vi "Generate Differential Drive Trajectory.vi"(8 "error in (no error)":errorcluster, 9 "Constraints":T1={"maxVoltage"=10.0, "maxVelocity"=5.0, "maxAccel"=10.0}, 10 "Constants":T2={"ks"=0.2, "kv"=0.18, "ka"=0.1, "trackwidth"=1.0}, 11 "Waypoints":T3[](array[typedef])=[{"Translation2d"={"x"=0.0, "y"=0.0}, "Rotation2d"={"Theta"=0.0}}, {"Translation2d"={"x"=1.0, "y"=1.0}, "Rotation2d"={"Theta"=1.0}}, {"Translation2d"={"x"=3.0, "y"=4.0}, "Rotation2d"={"Theta"=2.0}}]) -> (0 "error out":errorcluster, 2 "Total Time Seconds":dbl, 3 "states":T6[](array[typedef]))   [LabVIEW 2019]
uses:
  Typedef/Trajectory State.ctl
  Geometry/Typedef/Pose2d.ctl
  Geometry/Typedef/Translation2d.ctl
  Geometry/Typedef/Rotation2d.ctl
  Typedef/Differential Drive Constants.ctl
  Typedef/Differential Drive Constraints.ctl
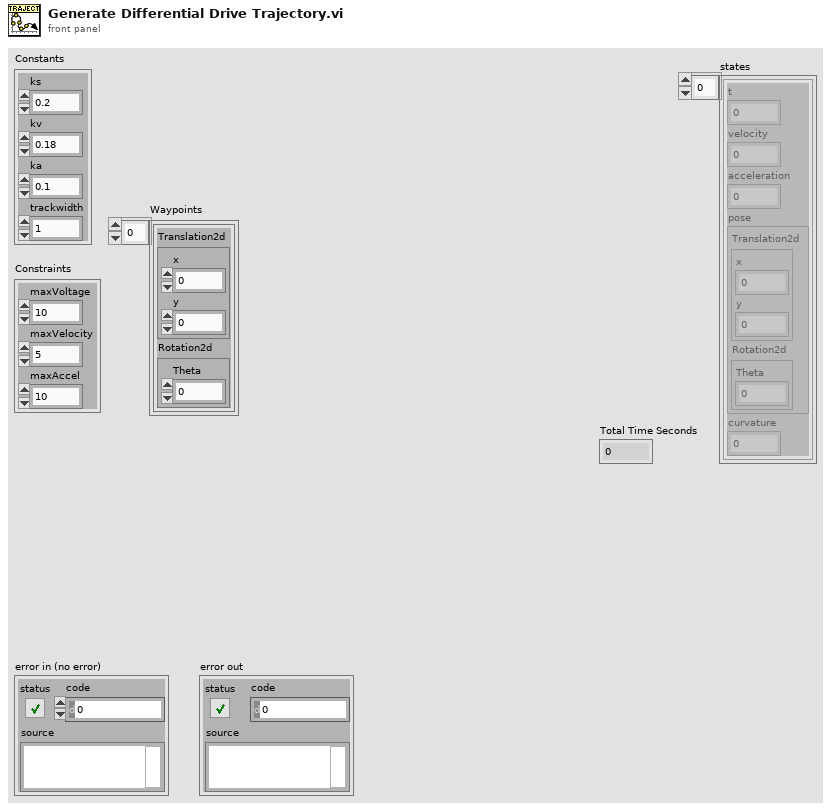
[diagram p1: front panel]
types:
  T1 = typedef "Differential Drive Constraints.ctl" = cluster{"maxVoltage":dbl, "maxVelocity":dbl, "maxAccel":dbl}
  T2 = typedef "Differential Drive Constants.ctl" = cluster{"ks":dbl, "kv":dbl, "ka":dbl, "trackwidth":dbl}
  T3 = typedef "Pose2d.ctl" = cluster{"Translation2d":T4, "Rotation2d":T5}
  T4 = typedef "Translation2d.ctl" = cluster{"x":dbl, "y":dbl}
  T5 = typedef "Rotation2d.ctl" = cluster{"Theta":dbl}
  T6 = typedef "Trajectory State.ctl" = cluster{"t":dbl, "velocity":dbl, "acceleration":dbl, "pose":T3, "curvature":dbl}
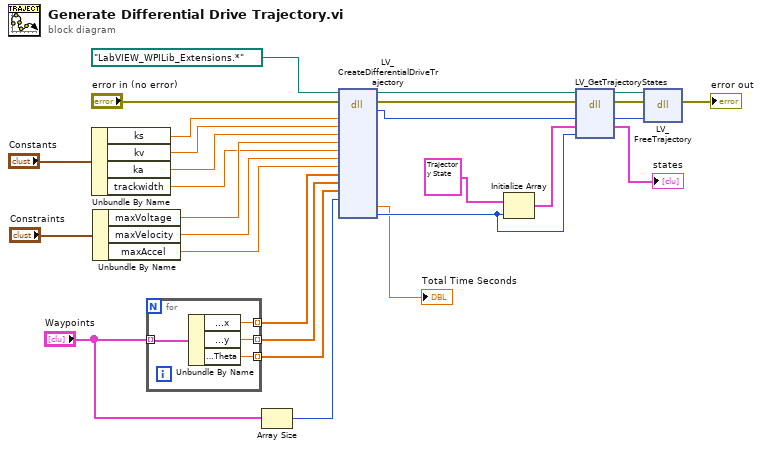
[diagram p0: block diagram]
diagram:
  n1 = Unbundle By Name("Constants") -> ("ks"=w15:dbl, "kv"=w16:dbl, "ka"=w17:dbl, "trackwidth"=w18:dbl)
  n2 = Unbundle By Name("Constraints") -> ("maxVoltage"=w20:dbl, "maxVelocity"=w21:dbl, "maxAccel"=w22:dbl)
  n3 = for {
    tunnel: "Waypoints" -> [w32] mode=indexing
    tunnel: [w31] -> w11 mode=indexing
    tunnel: [w30] -> w12 mode=indexing
    tunnel: [w29] -> w13 mode=indexing
    n4 = Unbundle By Name(w32) -> ("Translation2d.x"=w31:dbl, "Translation2d.y"=w30:dbl, "Rotation2d.Theta"=w29:dbl)
  }
  n5 = Array Size(array="Waypoints") -> (size(s)=w9:i32)
  n6 = dll-call lib="?" fn="LV_CreateDifferentialDriveTrajectory"(path in=path "LabVIEW_WPILib_Extensions.*", error in="error in (no error)", "ks"=w15, "kv"=w16, "ka"=w17, "maxVoltage"=w20, "trackwidth"=w18, "maxVelocity"=w21, "maxAccel"=w22, "waypoints_x"=w11, "waypoints_y"=w12, "waypoints_theta"=w13, "numPoints"=w9) -> (path out=w24:path, error out=w26:errorcluster, "return type"=w3:u64, "totalTimeSeconds"=→"Total Time Seconds":dbl, "trajectorySize"=w5:u32)  [unwired: 14 in]
  n7 = Initialize Array(T6 {"t"=0.0, "velocity"=0.0, "acceleration"=0.0, "pose"={"Translation2d"={"x"=0.0, "y"=0.0}, "Rotation2d"={"Theta"=0.0}}, "curvature"=0.0}, w5) -> (w4:T6[])
  n8 = dll-call lib="?" fn="LV_GetTrajectoryStates"(path in=w24, error in=w26, "handle"=w3, "states"=w4, "bufsize"=w5) -> (path out=w25:path, error out=w27:errorcluster, "handle"=w7:u64, "states"=→"states":T6[])  [unwired: 3 in]
  n9 = dll-call lib="?" fn="LV_FreeTrajectory"(path in=w25, error in=w27, "handle"=w7) -> (error out=→"error out":errorcluster)  [unwired: 3 in, 1 out]
